vi "Waveform to 2D Array.vi"   [LabVIEW 2012]
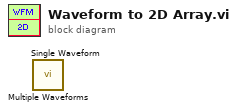
[diagram p0: block diagram]
diagram:
  n1 = call "Multiple Waveforms.vi"() -> ()  [unwired: 10 in, 2 out]
  n2 = call "Single Waveform.vi"() -> ()  [unwired: 10 in, 2 out]
